vi "Upload VASP File.vi"(8 "error in (no error)":errorcluster, 9 "Upload DOS?":bool, 10 "connection reference":T1, 11 "Directory to upload":path=path "C:/Users/Chris B/Documents/Ab Initio/Vasp Calculations/Batch4_20130519/1_Again") -> (0 "error out":errorcluster, 3 "IDs":T2)   [LabVIEW 2010]
uses:
  <vilib>/addons/database/Connection.llb/Conn ObjectReference.ctl
  <vilib>/Utility/error.llb/DialogType.ctl
  <vilib>/addons/database/Connection.llb/Conn Get Properties.vi
  <vilib>/addons/database/Connection.llb/DB Tools Open Connec (Path).vi
  <vilib>/Analysis/_algsub.llb/Real Vector Norm.vi
  <vilib>/Analysis/baseanly.llb/Real Dot Product.vi
  <vilib>/Utility/file.llb/Read From Spreadsheet File (string).vi
  <vilib>/addons/database/NI_Database_API.lvlib
  <vilib>/Analysis/NI_AALBase.lvlib
  <vilib>/Analysis/NI_AALPro.lvlib
panel:
  out "INCAR":bool
  out "INCAR ID":string
  in  "Show Errors?":bool
  out "README":bool
  out "# of atoms":i32
  out "CONTCAR":T3
  out "POSCAR":T3
  out "OUTCAR":bool
  out "DOSCAR":bool
  out "CONTCAR":bool
  out "POSCAR":bool
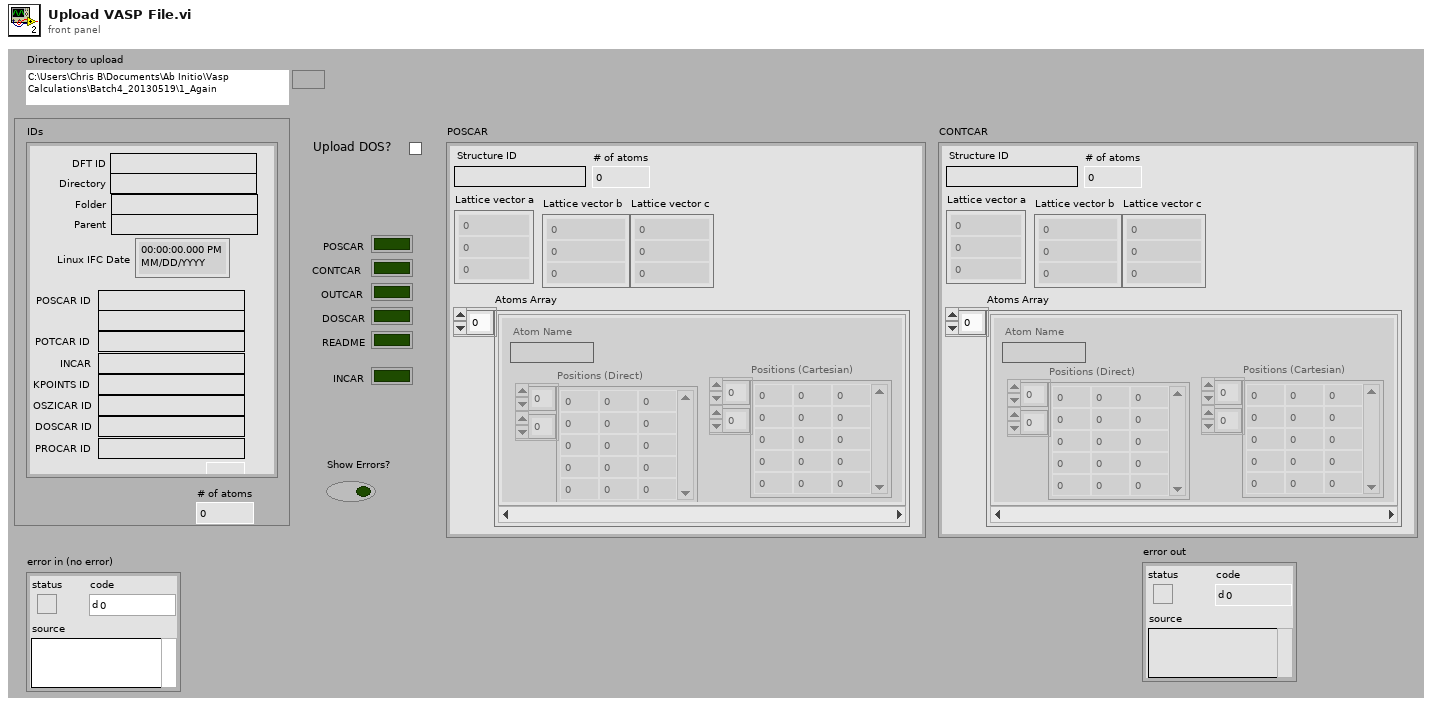
[diagram p1: front panel]
types:
  T1 = typedef "NI_Database_API.lvlib/Conn ObjectReference.ctl" = refnum<k1>
  T2 = cluster{"DFT ID":string, "Directory":string, "Folder":string, "Parent":string, "Linux IFC Date":timestamp, "POSCAR ID":string, "CONTCAR ID":string, "POTCAR ID":string, "INCAR":string, "KPOINTS ID":string, "OSZICAR ID":string, "DOSCAR ID":string, "PROCAR ID":string, "Calc time (Hrs)":dbl}
  T3 = cluster{"Structure ID":string, "Lattice vector a":dbl[], "Lattice vector b":dbl[], "Lattice vector c":dbl[], "Atoms Array":cluster{"Atom Name":string, "Positions (Direct)":dbl[][], "Positions (Cartesian)":dbl[][]}[], "# of atoms":i32}
  T4 = cluster{"Command":string, "Value":string, "Comment":string}[]
  T5 = cluster{"INCAR ID":string, "IBRION":string, "ISIF":string, "ISMEAR":string, "ISPIN":string, "Net Charge":i32}
  T6 = cluster{"INCAR ID":string, "Command":string, "Value":string, "Comment":string}
  T7 = typedef "DialogType.ctl" = u16
  T8 = cluster{"Structure Name":string, "Lattice vector a":dbl[], "Lattice vector b":dbl[], "Lattice vector c":dbl[], "Atoms Array":cluster{"Atom Name":string, "Positions (Direct)":dbl[][], "Positions (Cartesian)":dbl[][]}[], "# of atoms":i32}
  T9 = cluster{"MD5 message-digest":string, string, "name":string, "name":string, "Relaxation Time":timestamp, "Structure ID":string, "Structure ID":string, "MD5 message-digest":string, "INCAR ID":string, "MD5 message-digest":string, "MD5 message-digest":string, "MD5 message-digest":string, "MD5 message-digest":string, "Calc Time (Hrs)":dbl}
  T10 = cluster{"Atom Name":string, "Positions (Direct)":dbl[][], "Positions (Cartesian)":dbl[][]}[]
  T11 = cluster{"[0]":string, "[1]":string, "[2]":string, "[3]":string, "[4]":string, "[5]":string, "[6]":string, "[7]":string, "[8]":string, "[9]":string, "[10]":string, "[11]":string, "[12]":string, "[13]":string, "[14]":string, "[15]":string, "[16]":string, "[17]":string}
  T12 = cluster{"Structure ID":string, "Atom Name":string, "Numeric":dbl, "Numeric":dbl, "Numeric":dbl}
  T13 = cluster{"POTCAR ID":string, "trimmed string":string}
  T14 = cluster{"OSZICAR data":cluster{"Total Free Energy (eV)":dbl, "E0 at Sigma=0 (eV)":dbl, "dE (eV)":dbl, "Electronic Relaxation":dbl[][]}[], "Ionic Relaxation Energies Array (eV)":dbl[], "Bulk Formation Energies Array (eV)":dbl[]}
  T15 = cluster{"Final Energy (eV)":dbl, "Final Energy/atom (eV/atom)":dbl, "Total Formation Energy (eV)":dbl}
  T16 = cluster{"OSZICAR ID":string, "Final Energy (eV)":dbl, "Final Energy/atom (eV/atom)":dbl, "Total Formation Energy (eV)":dbl, i32}
  T17 = cluster{"Energy (eV)":dbl[], "Total DOS":dbl[], "Integrated DOS":dbl[]}
  T18 = cluster{"Fermi Level (eV)":dbl, "# States":dbl, "Density of Valence Band":dbl, "Density of Condution Band":dbl}
  T19 = cluster{"DOSCAR ID":string, "Energy (eV)":dbl[], "Total DOS":dbl[], "Integrated DOS":dbl[], void}
  T20 = cluster{"DOSCAR ID":string, i32, void, void, void}
  T21 = cluster{"DFT ID":string, "String":string, "String":string}
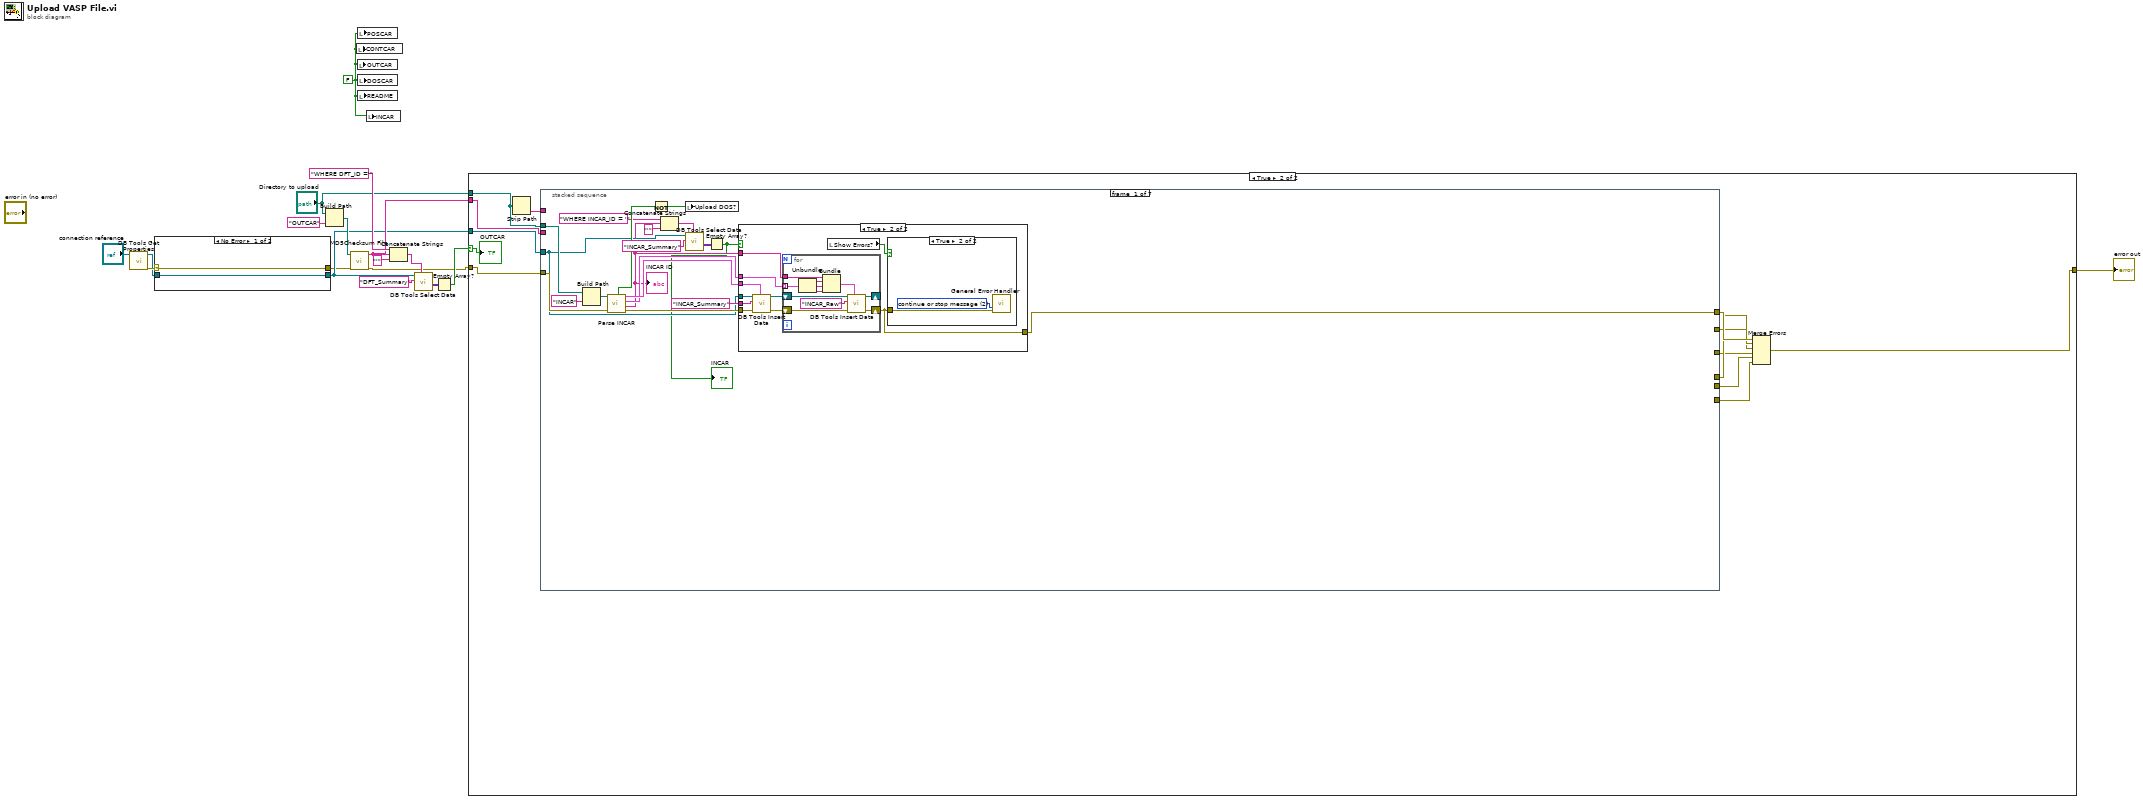
[diagram p0: block diagram]
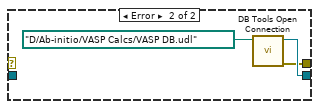
[diagram p2: hidden frame]
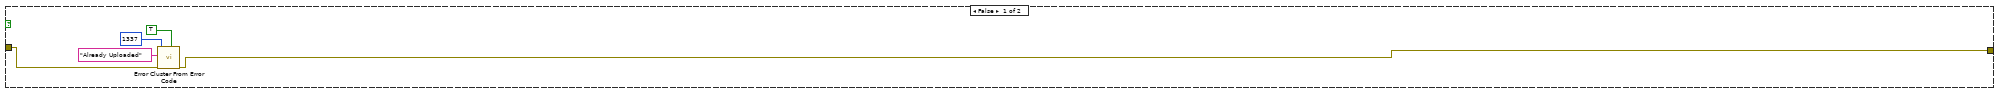
[diagram p3: hidden frame]
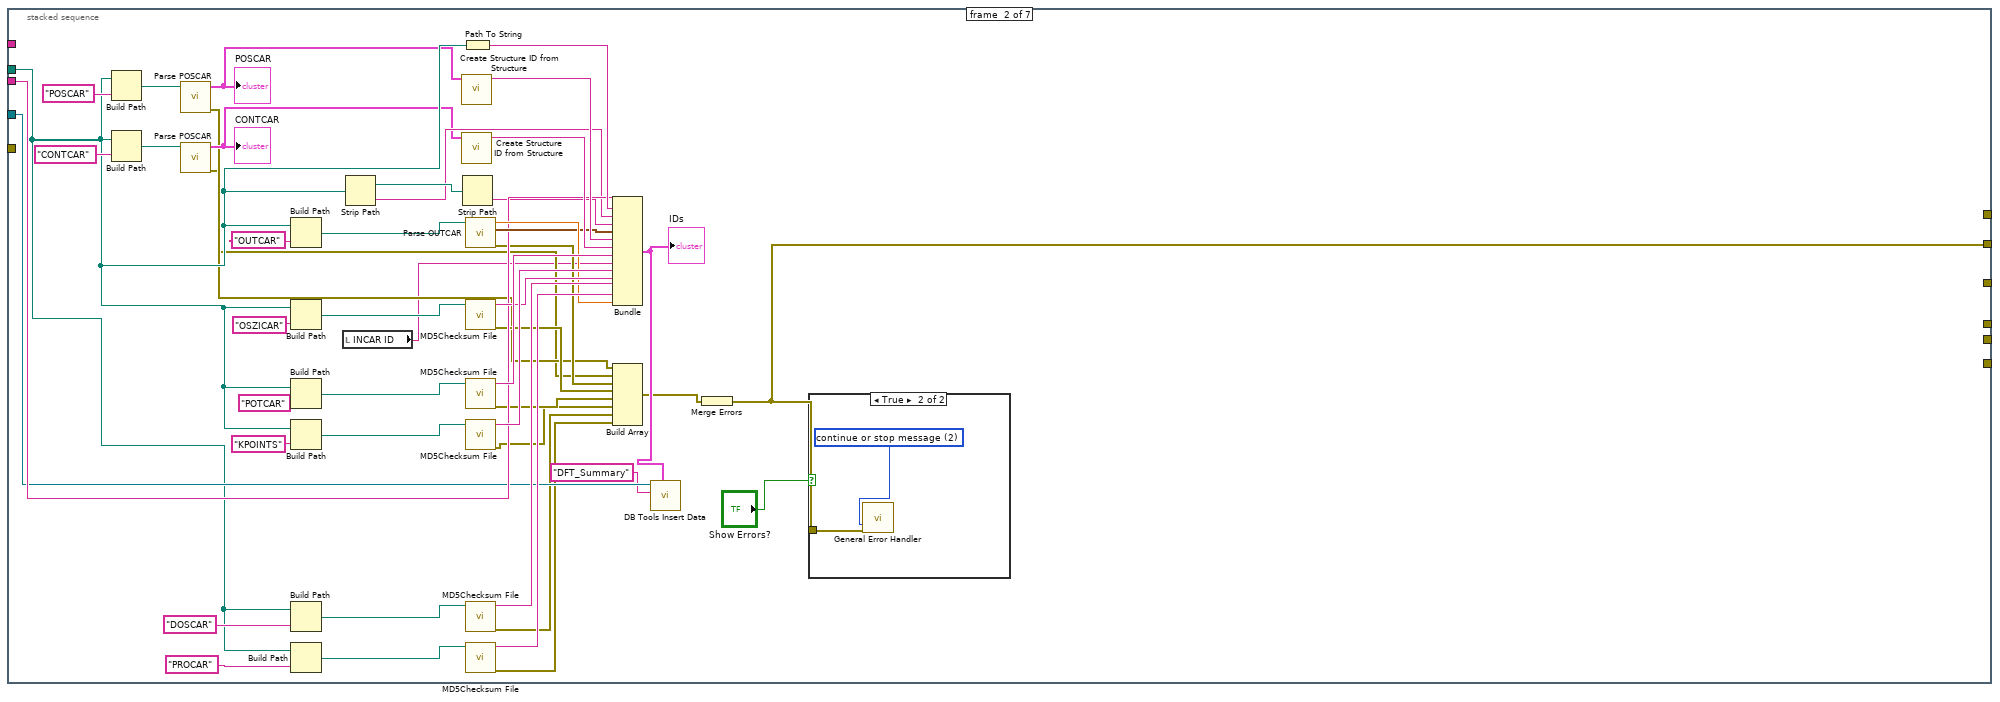
[diagram p6: hidden frame]
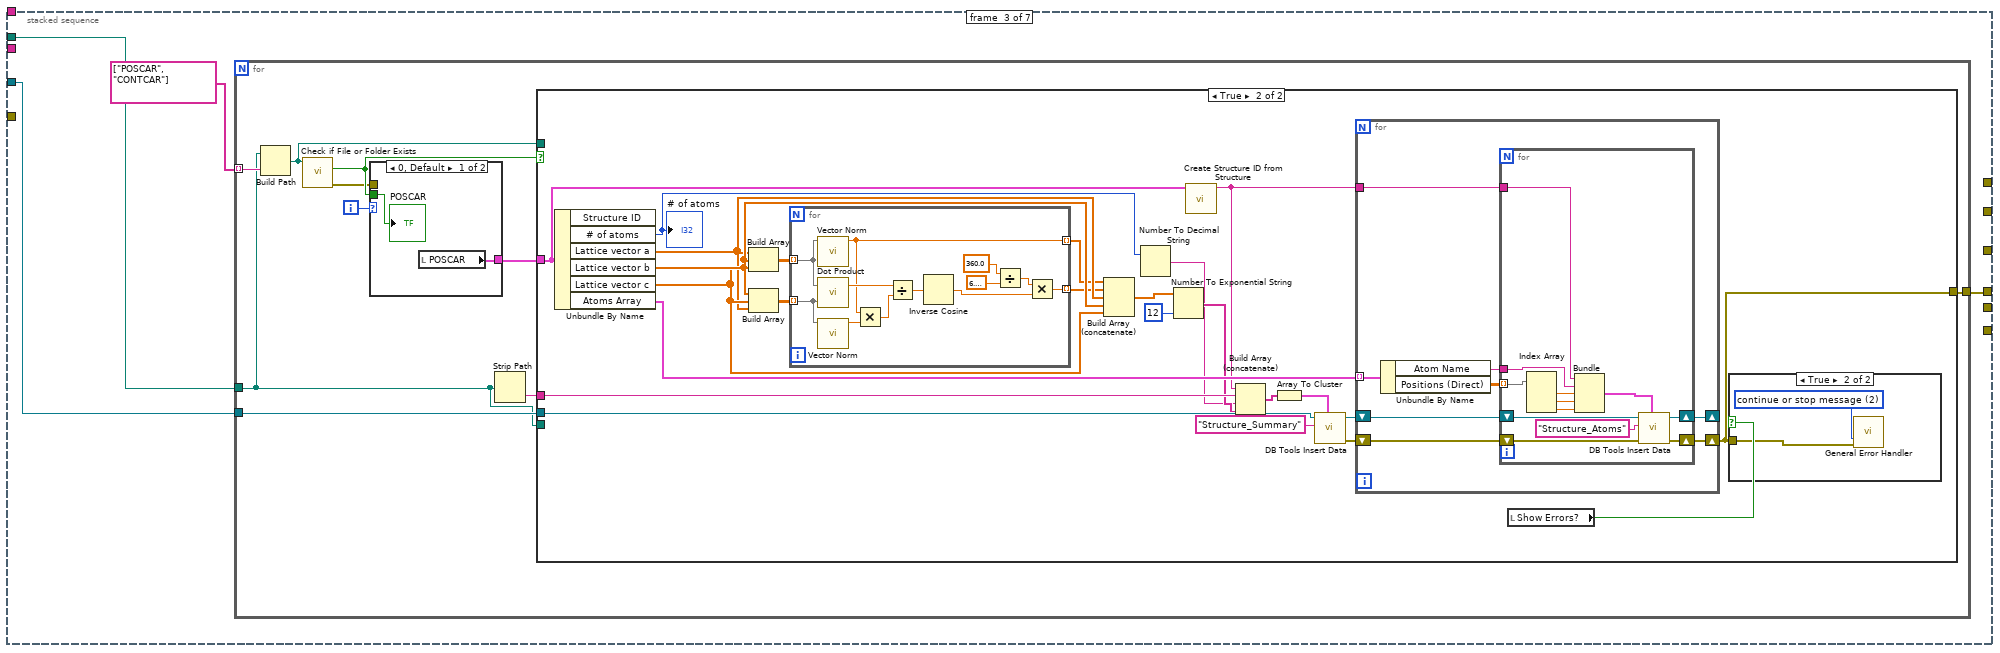
[diagram p8: hidden frame]
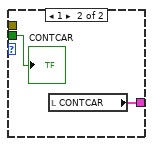
[diagram p11: hidden frame]
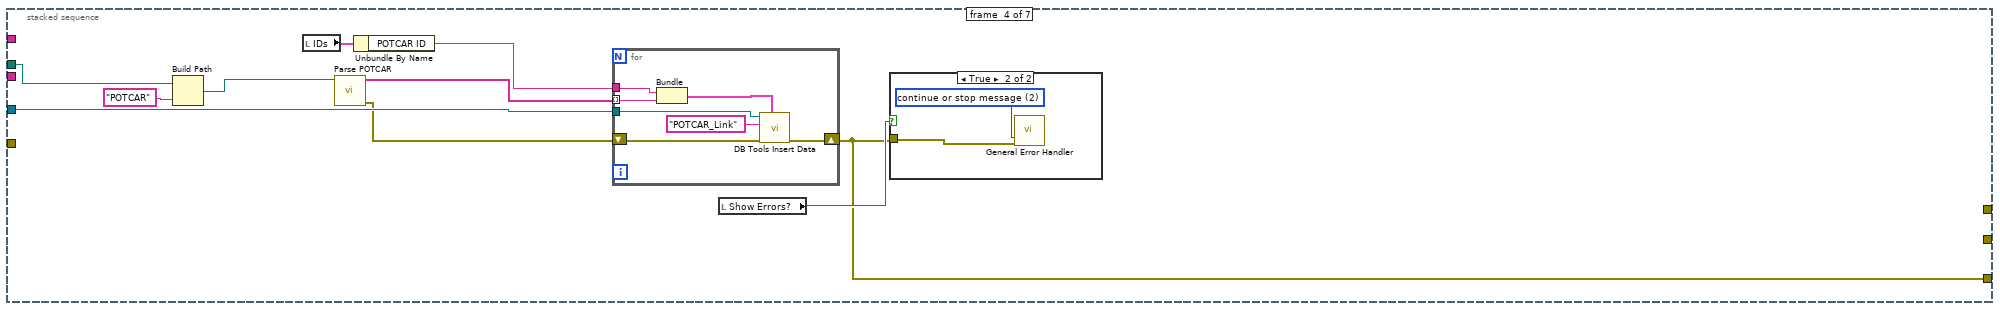
[diagram p12: hidden frame]
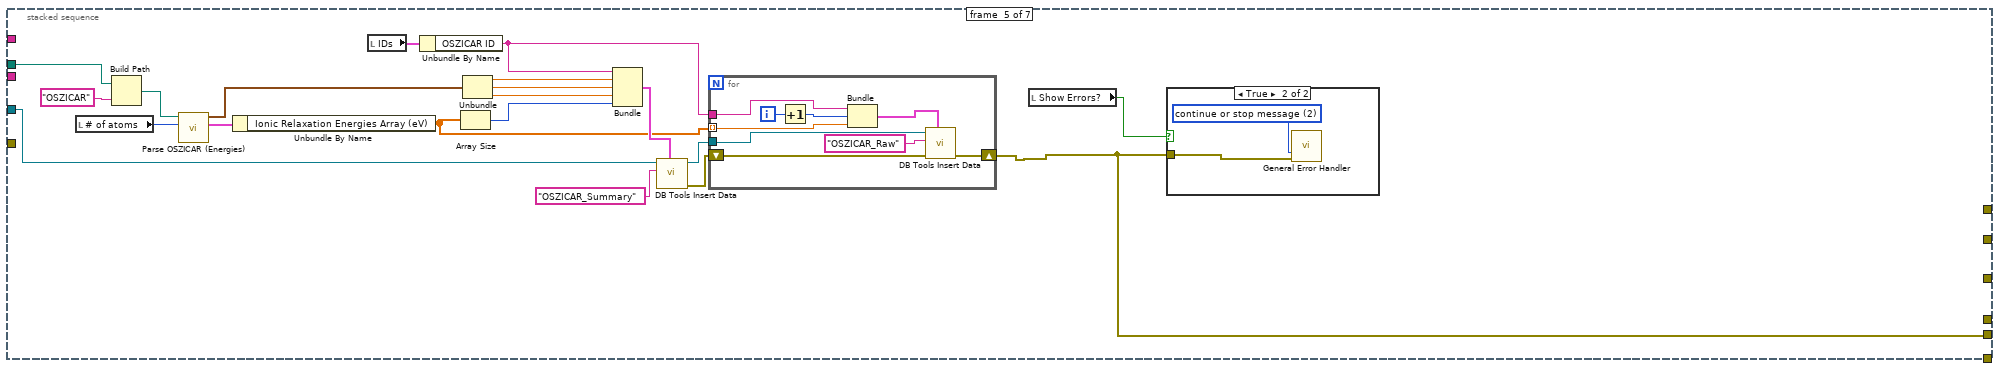
[diagram p14: hidden frame]
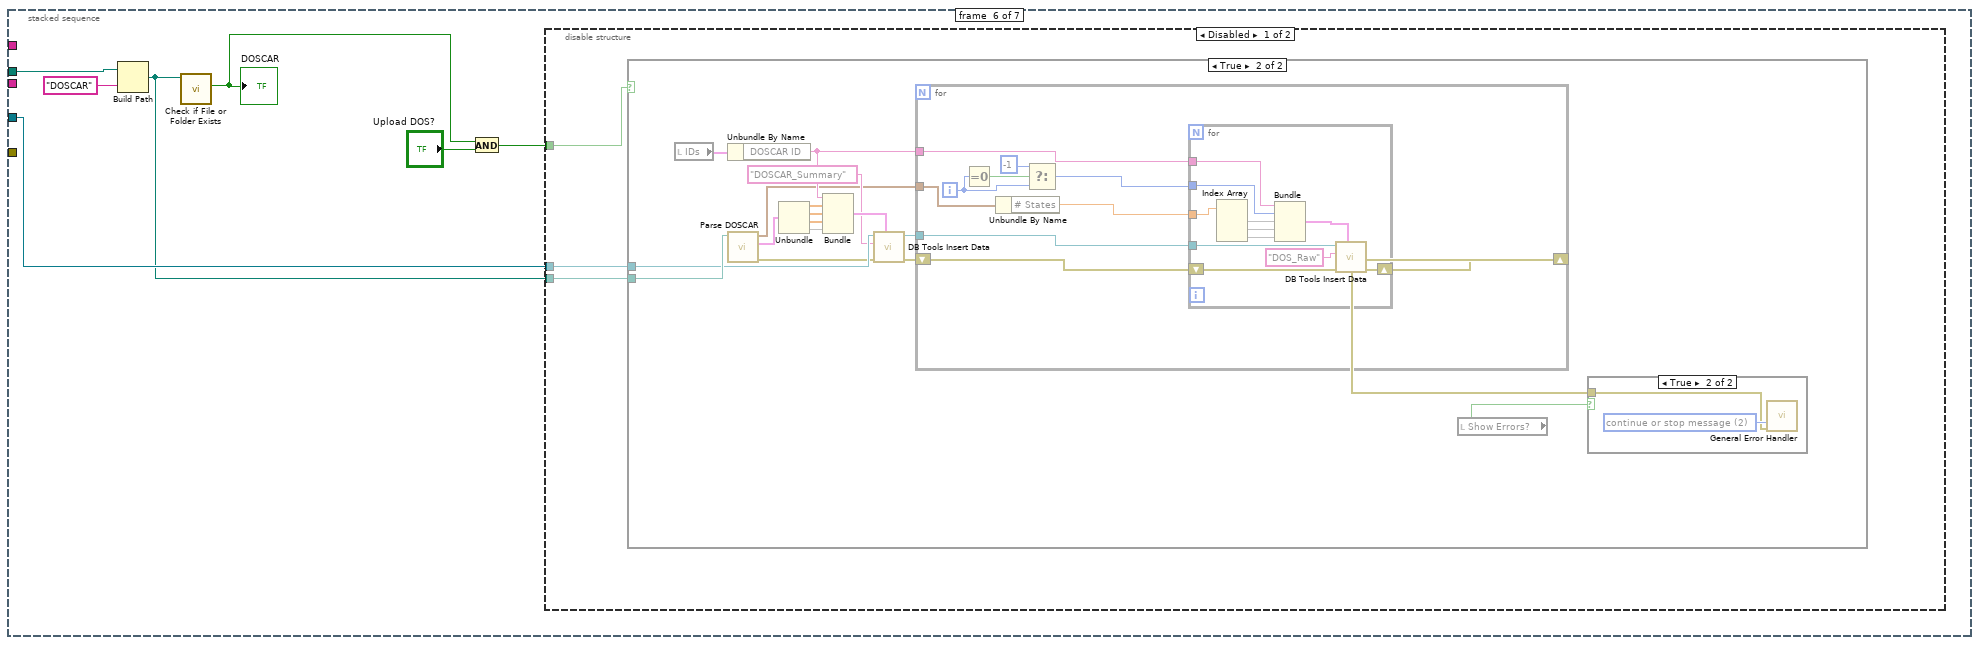
[diagram p16: hidden frame]
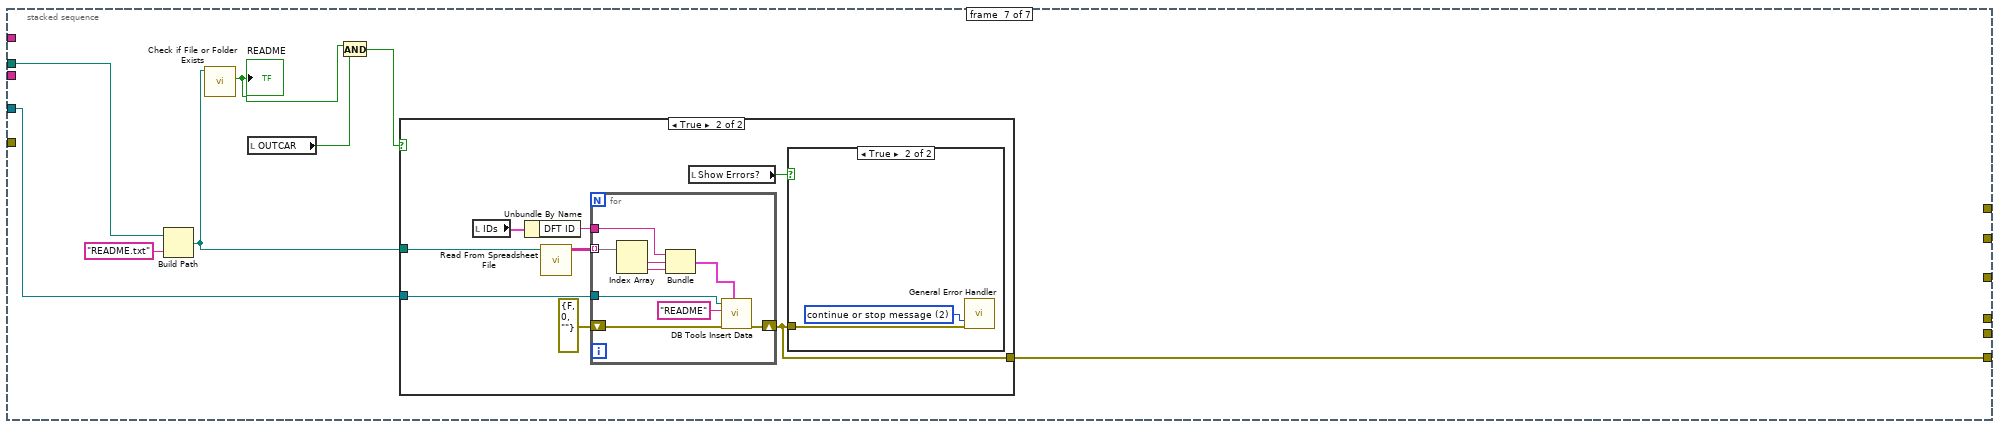
[diagram p20: hidden frame]
diagram:
  w1 = FALSE
  n1 = call-poly <vilib>:"DB Tools Get Properties.vi"("connection reference"="connection reference") -> ("error out"=w7:errorcluster, "connection reference out"=w6:T1)  [unwired: 4 in, 1 out]
  n2 = case shown="No Error" w7 {
    selector: w7 -> [w19 _]
    tunnel: w6 -> [w20 _]
    tunnel: [w20 w23] -> w5
    tunnel: [w19 w21] -> w4
    frame No Error {
    }
    frame Error {
      n3 = call-poly <vilib>:"DB Tools Open Connection.vi"("connection information"=path "D:/Ab-initio/VASP Calcs/VASP DB.udl" ("UDL")) -> ("error out"=w21:errorcluster, "connection reference"=w23:T1)  [unwired: 7 in]
    }
  }
  n4 = Build Path(base path="Directory to upload", name or relative path="OUTCAR") -> (appended path=w14:path)
  n5 = call <vilib>:"MD5Checksum File.vi"("error in (no error)"=w4, "Path"=w14) -> ("error out"=w9:errorcluster, "MD5 message-digest"=w12:string)  [unwired: 8 in]
  n6 = local write "CONTCAR"(w1) -> ()
  n7 = local write "OUTCAR"(w1) -> ()
  n8 = local write "POSCAR"(w1) -> ()
  n9 = local write "DOSCAR"(w1) -> ()
  n10 = local write "README"(w1) -> ()
  n11 = local write "INCAR"(w1) -> ()
  n12 = Concatenate Strings("WHERE DFT_ID ='" ("string"), w12, "'" ("string")) -> (w18:string)
  n13 = call <vilib>:"DB Tools Select Data.vi"("condition"=w18, "table"="DFT_Summary", "connection reference"=w5) -> ("data"=w3:variant[][])  [unwired: 3 in, 2 out]
  n14 = Empty Array?(array=w3) -> (empty?=w10:bool)
  n15 = case shown="True" w10 {
    selector: w10 -> [_ w37]
    tunnel: w12 -> [_ w40]
    tunnel: w5 -> [_ w39]
    tunnel: "Directory to upload" -> [_ w38]
    tunnel: w9 -> [w25 w36]
    tunnel: [w27 w29] -> w2
    frame False {
      n16 = call <vilib>:"Error Cluster From Error Code.vi"("is warning? (False)"=TRUE, "error in (no error)"=w25, "error message (\"\")"="Already Uploaded" ("error message (\"\")"), "error code (0)"=1337) -> ("error out"=w27:errorcluster)  [unwired: 5 in]
    }
    frame True {
      n17 = Strip Path(path=w38) -> (name=w41:string)  [unwired: 1 out]
      n18 = stacked-sequence {
        tunnel: w38 -> [w60 w104 w138 w220 w248 w267 w317]
        tunnel: w39 -> [w49 w105 w137 w214 w237 w266 w316]
        tunnel: w41 -> [_ _ _ _ _ _ _]
        tunnel: w40 -> [_ w106 _ _ _ _ _]
        tunnel: w36 -> [w51 _ _ _ _ _ _]
        tunnel: [w50 _ _ _ _ _ _] -> w35
        tunnel: [_ w85 _ _ _ _ _] -> w34
        tunnel: [_ _ w135 _ _ _ _] -> w33
        tunnel: [_ _ _ w211 _ _ _] -> w32
        tunnel: [_ _ _ _ w230 _ _] -> w31
        tunnel: [_ _ _ _ _ _ w311] -> w30
        frame #0 {
          n19 = Build Path(base path=w60, name or relative path="INCAR") -> (appended path=w58:path)
          n20 = call "Parse INCAR.vi"("error in (no error)"=w51, "INCAR File"=w58) -> ("error out"=w52:errorcluster, "INCAR ID"=w46:string, "INCAR Raw Commands"=w54:T4, "INCAR Summary"=w55:T5, "Allow Relaxation?"=w53:bool)  [unwired: 5 in]
          "INCAR ID" <- w46
          n21 = Not(x=w53) -> (.not. x?=w57:bool)
          n22 = Concatenate Strings("WHERE INCAR_ID = '" ("string"), w46, "'" ("string")) -> (w44:string)
          n23 = local write "Upload DOS?"(w57) -> ()
          n24 = call <vilib>:"DB Tools Select Data.vi"("condition"=w44, "table"="INCAR_Summary", "connection reference"=w49) -> ("data"=w43:variant[][])  [unwired: 3 in, 2 out]
          n25 = Empty Array?(array=w43) -> (empty?=w42:bool)
          "INCAR" <- w42
          n26 = case shown="True" w42 {
            tunnel: "INCAR_Summary" ("table") -> [_ w70]
            tunnel: w55 -> [_ w69]
            tunnel: w54 -> [_ w68]
            tunnel: w52 -> [w61 w67]
            tunnel: [w61 w64] -> w50
            tunnel: w49 -> [_ w63]
            tunnel: w46 -> [_ w62]
            frame False {
            }
            frame True {
              n27 = call <vilib>:"DB Tools Insert Data.vi"("data"=w69, "error in (no error)"=w67, "table"=w70, "connection reference"=w63) -> ("error out"=w65:errorcluster, "connection reference out"=w71:T1)  [unwired: 6 in]
              n28 = for {
                tunnel: w68 -> [w84] mode=indexing
                tunnel: w62 -> [w77]
                shift-right: [w82] -> _
                shift-left: w71 -> [w83]
                shift-right: [w75] -> w64
                shift-left: w65 -> [w74]
                n29 = Unbundle(w84) -> ("Command"=w81:string, "Value"=w80:string, "Comment"=w79:string)
                n30 = Bundle("INCAR ID"=w77, "Command"=w81, "Value"=w80, "Comment"=w79) -> (w78:T6)  [unwired: 1 in]
                n31 = call <vilib>:"DB Tools Insert Data.vi"("data"=w78, "error in (no error)"=w74, "table"="INCAR_Raw", "connection reference"=w83) -> ("error out"=w75:errorcluster, "connection reference out"=w82:T1)  [unwired: 6 in]
              }
              n32 = local read "Show Errors?"() -> (w66:bool)
              n33 = case shown="True" w66 {
                tunnel: w64 -> [_ w72]
                frame False {
                }
                frame True {
                  w73 = T7 2 items=["no dialog", "OK message", "continue or stop message", "OK message + warnings", "continue/stop + warnings"] ("type of dialog (OK msg:1)")
                  n34 = call <vilib>:"General Error Handler.vi"("type of dialog (OK msg:1)"=w73, "error in (no error)"=w72) -> ()  [unwired: 9 in, 5 out]
                }
              }
            }
          }
        }
        frame #1 {
          n35 = Build Path(base path=w104, name or relative path="POSCAR") -> (appended path=w126:path)
          n36 = Build Path(base path=w104, name or relative path="CONTCAR") -> (appended path=w125:path)
          n37 = call "Parse POSCAR.vi"("POSCAR File"=w126) -> ("error out"=w90:errorcluster, "Structure"=w92:T8)  [unwired: 7 in, 2 out]
          "POSCAR" <- w92
          n38 = call "Parse POSCAR.vi"("POSCAR File"=w125) -> ("error out"=w89:errorcluster, "Structure"=w91:T8)  [unwired: 7 in, 2 out]
          "CONTCAR" <- w91
          n39 = Build Path(base path=w104, name or relative path="OUTCAR") -> (appended path=w131:path)
          n40 = Build Path(base path=w104, name or relative path="OSZICAR") -> (appended path=w118:path)
          n41 = Build Path(base path=w104, name or relative path="POTCAR") -> (appended path=w129:path)
          n42 = Build Path(base path=w104, name or relative path="KPOINTS") -> (appended path=w119:path)
          n43 = Build Path(base path=w104, name or relative path="DOSCAR") -> (appended path=w112:path)
          n44 = Build Path(base path=w104, name or relative path="PROCAR") -> (appended path=w113:path)
          n45 = local read "INCAR ID"() -> (w86:string)
          n46 = Strip Path(path=w104) -> (stripped path=w103:path, name=w102:string)
          n47 = call "Create Structure ID from Structure.vi"("Structure"=w92) -> ("Structure ID"=w123:string)  [unwired: 10 in]
          n48 = call "Create Structure ID from Structure.vi"("Structure"=w91) -> ("Structure ID"=w122:string)  [unwired: 10 in]
          n49 = Path To String(path=w104) -> (string=w124:string)
          n50 = Strip Path(path=w103) -> (name=w101:string)  [unwired: 1 out]
          n51 = call "Parse OUTCAR.vi"("OUTCAR File"=w131) -> ("error out"=w93:errorcluster, "Relaxation Time"=w107:timestamp, "Calc Time (Hrs)"=w108:dbl)  [unwired: 8 in]
          n52 = call <vilib>:"MD5Checksum File.vi"("Path"=w118) -> ("error out"=w98:errorcluster, "MD5 message-digest"=w115:string)  [unwired: 9 in]
          n53 = call <vilib>:"MD5Checksum File.vi"("Path"=w129) -> ("error out"=w97:errorcluster, "MD5 message-digest"=w121:string)  [unwired: 9 in]
          n54 = call <vilib>:"MD5Checksum File.vi"("Path"=w119) -> ("error out"=w96:errorcluster, "MD5 message-digest"=w116:string)  [unwired: 9 in]
          n55 = call <vilib>:"MD5Checksum File.vi"("Path"=w112) -> ("error out"=w95:errorcluster, "MD5 message-digest"=w110:string)  [unwired: 9 in]
          n56 = call <vilib>:"MD5Checksum File.vi"("Path"=w113) -> ("error out"=w94:errorcluster, "MD5 message-digest"=w109:string)  [unwired: 9 in]
          n57 = Bundle("MD5 message-digest"=w106, w124, "name"=w102, "name"=w101, "Relaxation Time"=w107, "Structure ID"=w123, "Structure ID"=w122, "MD5 message-digest"=w121, "INCAR ID"=w86, "MD5 message-digest"=w116, "MD5 message-digest"=w115, "MD5 message-digest"=w110, "MD5 message-digest"=w109, "Calc Time (Hrs)"=w108) -> (w99:T9)  [unwired: 1 in]
          "IDs" <- w99
          n58 = Build Array(w90, w89, w93, w98, w97, w96, w95, w94) -> (w88:errorcluster[])
          n59 = call <vilib>:"DB Tools Insert Data.vi"("data"=w99, "table"="DFT_Summary", "connection reference"=w105) -> ()  [unwired: 7 in, 2 out]
          n60 = Merge Errors(w88) -> (w85:errorcluster)
          n61 = case shown="True" "Show Errors?" {
            tunnel: w85 -> [_ w134]
            frame False {
            }
            frame True {
              w133 = T7 2 items=["no dialog", "OK message", "continue or stop message", "OK message + warnings", "continue/stop + warnings"] ("type of dialog (OK msg:1)")
              n62 = call <vilib>:"General Error Handler.vi"("type of dialog (OK msg:1)"=w133, "error in (no error)"=w134) -> ()  [unwired: 9 in, 5 out]
            }
          }
        }
        frame #2 {
          n63 = for {
            tunnel: string[] ["POSCAR", "CONTCAR"] -> [w147] mode=indexing
            tunnel: w138 -> [w143]
            tunnel: w137 -> [w148]
            tunnel: [w139] -> w135
            i -> [w145]
            n64 = Build Path(base path=w143, name or relative path=w147) -> (appended path=w146:path)
            n65 = call <vilib>:"Check if File or Folder Exists.vi"("path"=w146) -> ("error out"=w140:errorcluster, "file or folder exists?"=w144:bool)  [unwired: 8 in, 1 out]
            n66 = case shown="0, Default" w145 {
              tunnel: w144 -> [w208 w210]
              tunnel: [w207 w209] -> w141
              tunnel: w140 -> [_ _]
              frame 0, Default {
                n67 = local read "POSCAR"() -> (w207:T3)
                "POSCAR" <- w208
              }
              frame 1 {
                n68 = local read "CONTCAR"() -> (w209:T3)
                "CONTCAR" <- w210
              }
            }
            n69 = Strip Path(path=w143) -> (name=w142:string)  [unwired: 1 out]
            n70 = case shown="True" w144 {
              tunnel: w148 -> [_ w172]
              tunnel: w143 -> [_ _]
              tunnel: w146 -> [_ _]
              tunnel: w142 -> [_ w171]
              tunnel: w141 -> [_ w154]
              tunnel: [_ w149] -> w139
              frame False {
              }
              frame True {
                n71 = Unbundle By Name(w154) -> ("# of atoms"=w150:i32, "Lattice vector a"=w167:dbl[], "Lattice vector b"=w169:dbl[], "Lattice vector c"=w168:dbl[], "Atoms Array"=w158:T10)  [unwired: 1 out]
                "# of atoms" <- w150
                n72 = Build Array(w167, w169, w168) -> (w170:dbl[][])
                n73 = Build Array(w169, w168, w167) -> (w166:dbl[][])
                n74 = for {
                  tunnel: w170 -> [w205] mode=indexing
                  tunnel: w166 -> [w204] mode=indexing
                  tunnel: [w200] -> w165 mode=indexing
                  tunnel: [w196] -> w164 mode=indexing
                  n75 = call-poly <vilib>:"Vector Norm.vi"("Input Vector"=w205) -> ("norm"=w200:dbl)  [unwired: 9 in, 1 out]
                  n76 = call-poly <vilib>:"Dot Product.vi"("Y Vector"=w204, "X Vector"=w205) -> ("X * Y"=w206:dbl)  [unwired: 1 out]
                  n77 = call-poly <vilib>:"Vector Norm.vi"("Input Vector"=w204) -> ("norm"=w203:dbl)  [unwired: 9 in, 1 out]
                  n78 = Multiply(x=w200, y=w203) -> (x*y=w202:dbl)
                  n79 = Divide(x=w206, y=w202) -> (x/y=w201:dbl)
                  n80 = Inverse Cosine(1:w201) -> (0:w197:dbl)
                  n81 = Divide(x=360.0, y=6.283185307179586) -> (x/y=w198:dbl)
                  n82 = Multiply(x=w198, y=w197) -> (x*y=w196:dbl)
                }
                n83 = Build Array (concatenate)(w165, w164, w167, w169, w168) -> (w163:dbl[])
                n84 = Number To Decimal String(number=w150) -> (decimal integer string=w151:string)  [unwired: 1 in]
                n85 = Number To Exponential String(number=w163, precision (6)=i16 12) -> (E-format string=w152:string[])  [unwired: 2 in]
                n86 = call "Create Structure ID from Structure.vi"("Structure"=w154) -> ("Structure ID"=w155:string)  [unwired: 10 in]
                n87 = Build Array (concatenate)(w155, w171, w151, w152) -> (w161:string[])
                n88 = Array To Cluster(array=w161) -> (cluster=w160:T11)
                n89 = call <vilib>:"DB Tools Insert Data.vi"("data"=w160, "table"="Structure_Summary", "connection reference"=w172) -> ("error out"=w157:errorcluster, "connection reference out"=w156:T1)  [unwired: 7 in]
                n90 = for {
                  tunnel: w158 -> [w182] mode=indexing
                  shift-right: [w179] -> w149
                  shift-left: w157 -> [w180]
                  shift-right: [w178] -> _
                  shift-left: w156 -> [w181]
                  tunnel: w155 -> [w175]
                  n91 = Unbundle By Name(w182) -> ("Atom Name"=w177:string, "Positions (Direct)"=w176:dbl[][])
                  n92 = for {
                    shift-right: [w193] -> w178
                    shift-left: w181 -> [w194]
                    shift-right: [w191] -> w179
                    shift-left: w180 -> [w192]
                    tunnel: w177 -> [w190]
                    tunnel: w176 -> [w188] mode=indexing
                    tunnel: w175 -> [w189]
                    n93 = Index Array(array=w188) -> (element #1=w187:dbl, element #2=w186:dbl, element #3=w185:dbl)  [unwired: 3 in]
                    n94 = Bundle("Structure ID"=w189, "Atom Name"=w190, "Numeric"=w187, "Numeric"=w186, "Numeric"=w185) -> (w184:T12)  [unwired: 1 in]
                    n95 = call <vilib>:"DB Tools Insert Data.vi"("data"=w184, "error in (no error)"=w192, "table"="Structure_Atoms", "connection reference"=w194) -> ("error out"=w191:errorcluster, "connection reference out"=w193:T1)  [unwired: 6 in]
                  }
                }
                n96 = local read "Show Errors?"() -> (w153:bool)
                n97 = case shown="True" w153 {
                  tunnel: w149 -> [_ w174]
                  frame False {
                  }
                  frame True {
                    w173 = T7 2 items=["no dialog", "OK message", "continue or stop message", "OK message + warnings", "continue/stop + warnings"] ("type of dialog (OK msg:1)")
                    n98 = call <vilib>:"General Error Handler.vi"("type of dialog (OK msg:1)"=w173, "error in (no error)"=w174) -> ()  [unwired: 9 in, 5 out]
                  }
                }
              }
            }
          }
        }
        frame #3 {
          n99 = Build Path(base path=w220, name or relative path="POTCAR") -> (appended path=w218:path)
          n100 = local read "IDs"() -> (w217:T2)
          n101 = call "Parse POTCAR.vi"("POTCAR File"=w218) -> ("error out"=w213:errorcluster, "POTCARs"=w216:string[])  [unwired: 9 in]
          n102 = Unbundle By Name(w217) -> ("POTCAR ID"=w215:string)
          n103 = for {
            tunnel: w216 -> [w229] mode=indexing
            tunnel: w215 -> [w228]
            tunnel: w214 -> [w225]
            shift-right: [w224] -> w211
            shift-left: w213 -> [w223]
            n104 = Bundle("POTCAR ID"=w228, "trimmed string"=w229) -> (w227:T13)  [unwired: 1 in]
            n105 = call <vilib>:"DB Tools Insert Data.vi"("data"=w227, "error in (no error)"=w223, "table"="POTCAR_Link", "connection reference"=w225) -> ("error out"=w224:errorcluster)  [unwired: 6 in, 1 out]
          }
          n106 = local read "Show Errors?"() -> (w212:bool)
          n107 = case shown="True" w212 {
            tunnel: w211 -> [_ w222]
            frame False {
            }
            frame True {
              w221 = T7 2 items=["no dialog", "OK message", "continue or stop message", "OK message + warnings", "continue/stop + warnings"] ("type of dialog (OK msg:1)")
              n108 = call <vilib>:"General Error Handler.vi"("type of dialog (OK msg:1)"=w221, "error in (no error)"=w222) -> ()  [unwired: 9 in, 5 out]
            }
          }
        }
        frame #4 {
          n109 = local read "# of atoms"() -> (w246:i32)
          n110 = Build Path(base path=w248, name or relative path="OSZICAR") -> (appended path=w247:path)
          n111 = call "Parse OSZICAR (Energies).vi"("# of Atoms"=w246, "OSZICAR File"=w247) -> ("OSZICAR Raw"=w244:T14, "Extracted Parameters"=w243:T15)  [unwired: 6 in, 2 out]
          n112 = Unbundle By Name(w244) -> ("Ionic Relaxation Energies Array (eV)"=w234:dbl[])
          n113 = local read "IDs"() -> (w245:T2)
          n114 = Unbundle By Name(w245) -> ("OSZICAR ID"=w233:string)
          n115 = Array Size(array=w234) -> (size(s)=w239:i32)
          n116 = Unbundle(w243) -> ("Final Energy (eV)"=w242:dbl, "Final Energy/atom (eV/atom)"=w241:dbl, "Total Formation Energy (eV)"=w240:dbl)
          n117 = Bundle("OSZICAR ID"=w233, "Final Energy (eV)"=w242, "Final Energy/atom (eV/atom)"=w241, "Total Formation Energy (eV)"=w240, w239) -> (w238:T16)  [unwired: 1 in]
          n118 = call <vilib>:"DB Tools Insert Data.vi"("data"=w238, "table"="OSZICAR_Summary", "connection reference"=w237) -> ("error out"=w235:errorcluster, "connection reference out"=w236:T1)  [unwired: 7 in]
          n119 = for {
            tunnel: w236 -> [w260]
            shift-right: [w258] -> w230
            shift-left: w235 -> [w257]
            tunnel: w234 -> [w253] mode=indexing
            tunnel: w233 -> [w254]
            i -> [w256]
            n120 = Increment(x=w256) -> (x+1=w255:i32)
            n121 = Bundle("OSZICAR ID"=w254, w255, w253) -> (w252:cluster{"OSZICAR ID":string, i32, dbl})  [unwired: 1 in]
            n122 = call <vilib>:"DB Tools Insert Data.vi"("data"=w252, "error in (no error)"=w257, "table"="OSZICAR_Raw", "connection reference"=w260) -> ("error out"=w258:errorcluster)  [unwired: 6 in, 1 out]
          }
          n123 = local read "Show Errors?"() -> (w231:bool)
          n124 = case shown="True" w231 {
            tunnel: w230 -> [_ w251]
            frame False {
            }
            frame True {
              w250 = T7 2 items=["no dialog", "OK message", "continue or stop message", "OK message + warnings", "continue/stop + warnings"] ("type of dialog (OK msg:1)")
              n125 = call <vilib>:"General Error Handler.vi"("type of dialog (OK msg:1)"=w250, "error in (no error)"=w251) -> ()  [unwired: 9 in, 5 out]
            }
          }
        }
        frame #5 {
          n126 = Build Path(base path=w267, name or relative path="DOSCAR") -> (appended path=w264:path)
          n127 = call <vilib>:"Check if File or Folder Exists.vi"("path"=w264) -> ("file or folder exists?"=w262:bool)  [unwired: 8 in, 2 out]
          "DOSCAR" <- w262
          n128 = And(x=w262, y="Upload DOS?") -> (x .and. y?=w263:bool)
          n129 = disable-structure shown="Disabled" {
            disable-tunnel: w266 -> [w270 _]
            disable-tunnel: w264 -> [w269 _]
            disable-tunnel: w263 -> [w268 _]
            frame Disabled {
              n130 = case shown="True" w268 {
                tunnel: w270 -> [_ w278]
                tunnel: w269 -> [_ w287]
                frame False {
                }
                frame True {
                  n131 = local read "IDs"() -> (w286:T2)
                  n132 = Unbundle By Name(w286) -> ("DOSCAR ID"=w284:string)
                  n133 = call "Parse DOSCAR.vi"("Path"=w287) -> ("error out"=w273:errorcluster, "Total DOS"=w285:T17, "DOS Summary"=w274:T18)  [unwired: 7 in, 1 out]
                  n134 = Unbundle(w285) -> (w283:dbl[], w282:dbl[], w280:dbl[], w281)
                  n135 = Bundle("DOSCAR ID"=w284, "Energy (eV)"=w283, "Total DOS"=w282, "Integrated DOS"=w280, w281) -> (w279:T19)  [unwired: 1 in]
                  n136 = call <vilib>:"DB Tools Insert Data.vi"("data"=w279, "error in (no error)"=w273, "table"="DOSCAR_Summary", "connection reference"=w278) -> ("error out"=w276:errorcluster, "connection reference out"=w277:T1)  [unwired: 6 in]
                  n137 = for {
                    tunnel: w277 -> [w297]
                    tunnel: w284 -> [w298]
                    shift-right: [w296] -> w272
                    shift-left: w276 -> [w295]
                    tunnel: w274 -> [w294]
                    i -> [w291]
                    n138 = Equal To 0?(x=w291) -> (x = 0?=w299:bool)
                    n139 = Unbundle By Name(w294) -> ("# States"=w293:dbl)
                    n140 = Select(t=-1, s=w299, f=w291) -> (s? t:f=w290:i32)
                    n141 = for {
                      tunnel: w298 -> [w308]
                      tunnel: w290 -> [w307]
                      tunnel: w293 -> [w306]
                      tunnel: w297 -> [w309]
                      shift-right: [w301] -> w296
                      shift-left: w295 -> [w300]
                      n142 = Index Array(array=w306) -> (element #1=w305, element #2=w304, element #3=w303)  [unwired: 3 in]
                      n143 = Bundle("DOSCAR ID"=w308, w307, w305, w304, w303) -> (w302:T20)  [unwired: 1 in]
                      n144 = call <vilib>:"DB Tools Insert Data.vi"("data"=w302, "error in (no error)"=w300, "table"="DOS_Raw", "connection reference"=w309) -> ("error out"=w301:errorcluster)  [unwired: 6 in, 1 out]
                    }
                  }
                  n145 = local read "Show Errors?"() -> (w271:bool)
                  n146 = case shown="True" w271 {
                    tunnel: w272 -> [_ w288]
                    frame False {
                    }
                    frame True {
                      w289 = T7 2 items=["no dialog", "OK message", "continue or stop message", "OK message + warnings", "continue/stop + warnings"] ("type of dialog (OK msg:1)")
                      n147 = call <vilib>:"General Error Handler.vi"("type of dialog (OK msg:1)"=w289, "error in (no error)"=w288) -> ()  [unwired: 9 in, 5 out]
                    }
                  }
                }
              }
            }
            frame Enabled {
            }
          }
        }
        frame #6 {
          n148 = Build Path(base path=w317, name or relative path="README.txt") -> (appended path=w315:path)
          n149 = call <vilib>:"Check if File or Folder Exists.vi"("path"=w315) -> ("file or folder exists?"=w314:bool)  [unwired: 8 in, 2 out]
          "README" <- w314
          n150 = local read "OUTCAR"() -> (w312:bool)
          n151 = And(x=w314, y=w312) -> (x .and. y?=w313:bool)
          n152 = case shown="True" w313 {
            tunnel: w316 -> [_ w323]
            tunnel: w315 -> [_ w321]
            tunnel: [_ w319] -> w311
            frame False {
            }
            frame True {
              n153 = local read "IDs"() -> (w326:T2)
              n154 = Unbundle By Name(w326) -> ("DFT ID"=w324:string)
              n155 = call-poly <vilib>:"Read From Spreadsheet File.vi"("file path (dialog if empty)"=w321) -> ("all rows"=w325:string[][])  [unwired: 6 in, 4 out]
              n156 = for {
                tunnel: w325 -> [w337] mode=indexing
                tunnel: w324 -> [w336]
                tunnel: w323 -> [w332]
                shift-right: [w331] -> w319
                shift-left: errorcluster {"status"=FALSE, "code"=0, "source"=""} ("error out") -> [w330]
                n157 = Index Array(array=w337) -> (element #1=w335:string, element #2=w334:string)  [unwired: 2 in]
                n158 = Bundle("DFT ID"=w336, "String"=w335, "String"=w334) -> (w333:T21)  [unwired: 1 in]
                n159 = call <vilib>:"DB Tools Insert Data.vi"("data"=w333, "error in (no error)"=w330, "table"="README", "connection reference"=w332) -> ("error out"=w331:errorcluster)  [unwired: 6 in, 1 out]
              }
              n160 = local read "Show Errors?"() -> (w320:bool)
              n161 = case shown="True" w320 {
                tunnel: w319 -> [_ w327]
                frame False {
                }
                frame True {
                  w328 = T7 2 items=["no dialog", "OK message", "continue or stop message", "OK message + warnings", "continue/stop + warnings"] ("type of dialog (OK msg:1)")
                  n162 = call <vilib>:"General Error Handler.vi"("type of dialog (OK msg:1)"=w328, "error in (no error)"=w327) -> ()  [unwired: 9 in, 5 out]
                }
              }
            }
          }
        }
      }
      n163 = Merge Errors(w35, w34, w33, w32, w31, w30) -> (w29:errorcluster)
      "OUTCAR" <- w37
    }
  }
  "error out" <- w2
